vi "Lookup Group.vi"(8 "error in (no error)":errorcluster, 10 "Group Name":string, 11 "Cluster in":refnum<class "Cluster Config.lvclass">) -> (0 "error out":errorcluster, 1 "Node":refnum<class "Node Config.lvclass">, 2 "Group":refnum<class "Group Config.lvclass">, 3 "Cluster out":refnum<class "Cluster Config.lvclass">)   [LabVIEW 2020, in "VolatusConfig.lvlib" / "Cluster Config.lvclass"]
uses:
  Cluster Config.lvclass
  C:/dev/lv20CE/relink/lv-volatus/VolatusConfig/VolatusConfigElement/VolatusConfigElement.lvclass
  Node/Node Config.lvclass
  Group/Group Config.lvclass
  Meta Type.ctl
  VolatusConfigElement/VolatusConfigElement.lvclass/VolatusConfigElement.ctl
  VolatusConfigElement/Element.vi
  lv-cdm/CDM-Config/Config Lookup/Match Meta.vi
  lv-cdm/CDM-Config/Config Element/Owner.vi
  lv-cdm/CDM-Config/Config Manager/Lookup Descendant.vi
  lv-cdm/CDM-Config/Config Filter/Config Lookup.lvclass
  Cluster Config.lvclass/Cluster Config.ctl
  VolatusConfigElement/VolatusConfigElement.lvclass
  VolatusConfig.lvlib
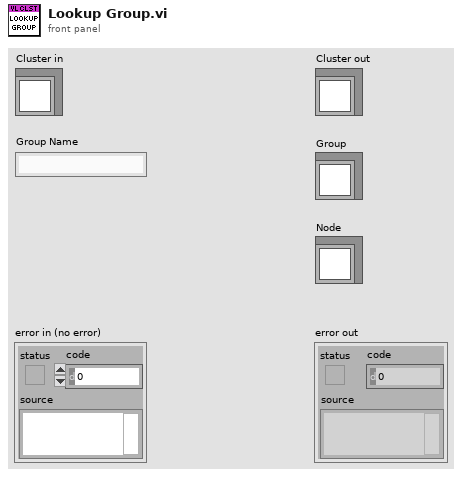
[diagram p1: front panel]
types:
  T1 = typedef "VolatusConfig.lvlib/Meta Type.ctl" = enum16{"UNKNOWN", "VL_System", "VL_Cluster", "VL_Node", "VL_Task", "VL_Group", "VL_Channel", "VL_Task_List", "VL_Scaling", "VL_Sensor", "VL_Sensor_List", "VL_Scale"}
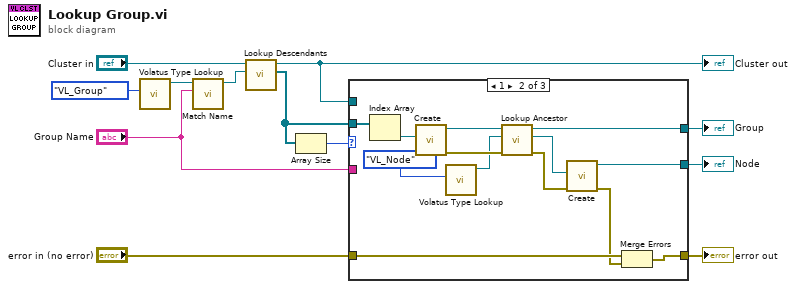
[diagram p0: block diagram]
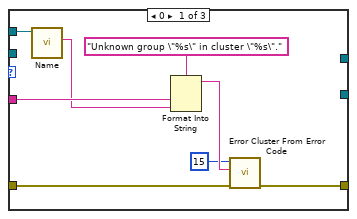
[diagram p2: hidden frame]
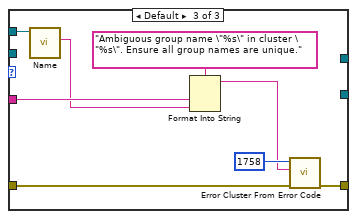
[diagram p3: hidden frame]
diagram:
  n1 = call "Volatus Type Lookup.vi"("Meta Type"=Meta_Type."VL_Group") -> ("Config Lookup out"=w11:refnum<class "Config Lookup.lvclass">)  [unwired: 9 in, 1 out]
  n2 = call "Match Name.vi"("Name"="Group Name", "Config Lookup (New)"=w11) -> ("Config Lookup out"=w10:refnum<class "Config Lookup.lvclass">)  [unwired: 8 in, 1 out]
  n3 = call "Lookup Descendants.vi"("Lookup"=w10, "VolatusConfigElement in"="Cluster in") -> ("Descendants"=w7:refnum<class "Config Element.lvclass">[], "VolatusConfigElement out"=w1:refnum<class "Cluster Config.lvclass">)  [unwired: 7 in, 1 out]
  "Cluster out" <- w1
  n4 = Array Size(array=w7) -> (size(s)=w8:i32)
  n5 = case shown="1" w8 {
    tunnel: w7 -> [_ w32 _]
    tunnel: [_ w29 _] -> w6
    tunnel: [_ w24 _] -> w5
    tunnel: "error in (no error)" -> [w19 w23 w40]
    tunnel: [w20 w21 w41] -> w3
    tunnel: "Group Name" -> [w16 _ w36]
    tunnel: w1 -> [w18 _ w35]
    frame 0 {
      n6 = call "Name.vi"("VolatusConfigElement in"=w18) -> ("Name"=w15:string)  [unwired: 8 in, 2 out]
      n7 = Format Into String(format string="Unknown group \"%s\" in cluster \"%s\".", w16, w15) -> (resulting string=w14:string)  [unwired: 2 in, 1 out]
      n8 = call <vilib>:"Error Cluster From Error Code.vi"("error in (no error)"=w19, "error message (\"\")"=w14, "error code (0)"=15) -> ("error out"=w20:errorcluster)  [unwired: 6 in]
    }
    frame 1 {
      n9 = Index Array(array=w32) -> (element=w31:refnum<class "Config Element.lvclass">)  [unwired: 1 in]
      n10 = call "Create.vi"("Element"=w31) -> ("error out"=w33:errorcluster, "Group out"=w30:refnum<class "Group Config.lvclass">)  [unwired: 9 in]
      n11 = call "Volatus Type Lookup.vi"("Meta Type"=Meta_Type."VL_Node") -> ("Config Lookup out"=w27:refnum<class "Config Lookup.lvclass">)  [unwired: 9 in, 1 out]
      n12 = call "Lookup Ancestor.vi"("error in (no error)"=w33, "Lookup"=w27, "VolatusConfigElement in"=w30) -> ("error out"=w25:errorcluster, "Ancestor"=w26:refnum<class "Config Element.lvclass">, "VolatusConfigElement out"=w29:refnum<class "Group Config.lvclass">)  [unwired: 6 in]
      n13 = call "Create.vi"("error in (no error)"=w25, "Element"=w26) -> ("error out"=w22:errorcluster, "Node out"=w24:refnum<class "Node Config.lvclass">)  [unwired: 8 in]
      n14 = Merge Errors(w23, w22) -> (w21:errorcluster)
    }
    frame Default {
      n15 = call "Name.vi"("VolatusConfigElement in"=w35) -> ("Name"=w34:string)  [unwired: 8 in, 2 out]
      n16 = Format Into String(format string="Ambiguous group name \"%s\" in cluster \"%s\". Ensure all group names are unique.", w36, w34) -> (resulting string=w38:string)  [unwired: 2 in, 1 out]
      n17 = call <vilib>:"Error Cluster From Error Code.vi"("error in (no error)"=w40, "error message (\"\")"=w38, "error code (0)"=1758) -> ("error out"=w41:errorcluster)  [unwired: 6 in]
    }
  }
  "error out" <- w3
  "Node" <- w5
  "Group" <- w6
